vi "getCoordsFromROI.vi"(0 "ROI":T1) -> (1 "y2":i32, 2 "x2":i32, 3 "y1":i32, 4 "x1":i32)   [LabVIEW 2015]
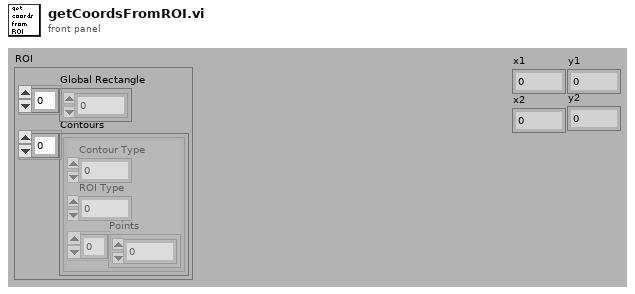
[diagram p1: front panel]
types:
  T1 = cluster{"Global Rectangle":i32[], "Contours":cluster{"Contour Type":u32, "ROI Type":u32, "Points":i32[]}[]}
  T2 = cluster{"Contour Type":u32, "ROI Type":u32, "Points":i32[]}[]
  T3 = cluster{"Contour Type":u32, "ROI Type":u32, "Points":i32[]}
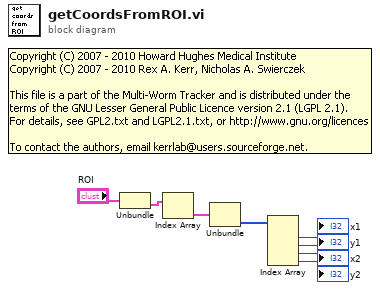
[diagram p0: block diagram]
diagram:
  n1 = Unbundle("ROI") -> ("Contours"=w7:T2)  [unwired: 1 out]
  n2 = Index Array(array=w7) -> (element=w6:T3)  [unwired: 1 in]
  n3 = Unbundle(w6) -> ("Points"=w5:i32[])  [unwired: 2 out]
  n4 = Index Array(array=w5) -> (element #1=→"x1":i32, element #2=→"y1":i32, element #3=→"x2":i32, element #4=→"y2":i32)  [unwired: 4 in]
